vi "Get Path.vi"(8 "error in":errorcluster, 10 "dir":string, 11 "path":path) -> (0 "error out":errorcluster, 2 "file or folder exists?":bool, 3 "dup path":path)   [LabVIEW 2014]
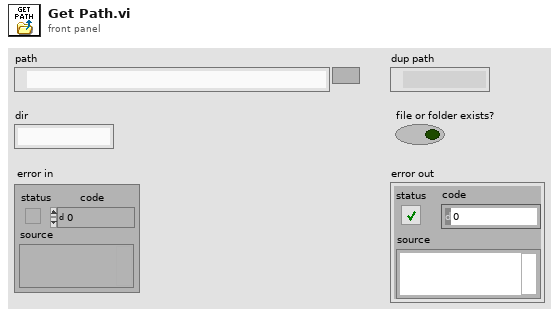
[diagram p1: front panel]
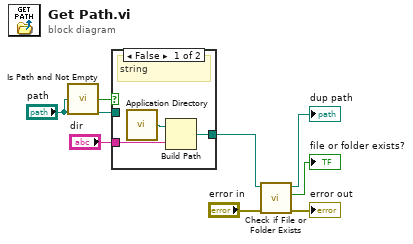
[diagram p0: block diagram]
diagram:
  n1 = call <vilib>:"Is Path and Not Empty.vi"("path"="path") -> ("Is Path and Not Empty?"=w1:bool)  [unwired: 4 in]
  n2 = case shown="False" w1 {
    tunnel: "path" -> [_ w12]
    tunnel: [w9 w12] -> w4
    tunnel: "dir" -> [w10 _]
    frame False {
      # "string"
      n3 = call <vilib>:"Application Directory.vi"() -> ("Application Directory"=w11:path)
      n4 = Build Path(base path=w11, name or relative path=w10) -> (appended path=w9:path)
    }
    frame True {
      # "path"
    }
  }
  n5 = call <vilib>:"Check if File or Folder Exists.vi"("error in (no error)"="error in", "path"=w4) -> ("error out"=→"error out":errorcluster, "file or folder exists?"=→"file or folder exists?":bool, "dup path"=→"dup path":path)  [unwired: 7 in]
